vi "Upgrade to Secure Server VISA Socket.vi"(7 "immutable TLS Configuration":refnum<k36>, 8 "error in (no error)":errorcluster, 9 "timeout (5000ms)":i32=5000, 11 "VISA TCP Socket in":refnum<class "VISA TCP.lvclass">) -> (0 "error out":errorcluster, 2 "client certificate chain":cluster{"certificate":u8[]}[](array[cluster]), 3 "Secure Server VISA Socket out":refnum<class "VISA TCP.lvclass">)   [LabVIEW 2020, in "Secure Sockets Addon.lvlib"]
doc: "Upgrades a Server VISA TCP Socket to use TLS."
uses:
  Secure Sockets Addon.lvlib
  <vilib>/MediaMongrels Ltd/WebSockets/Sockets/VISA TCP Socket/VISA TCP.lvclass
  <vilib>/MediaMongrels Ltd/WebSockets/Sockets/VISA TCP Socket/VISA TCP.lvclass/VISA TCP.ctl
  <vilib>/MediaMongrels Ltd/WebSockets/Sockets/VISA TCP Socket/Read TCP Refnum.vi
  <vilib>/MediaMongrels Ltd/WebSockets/Sockets/VISA TCP Socket/Write TCP Refnum.vi
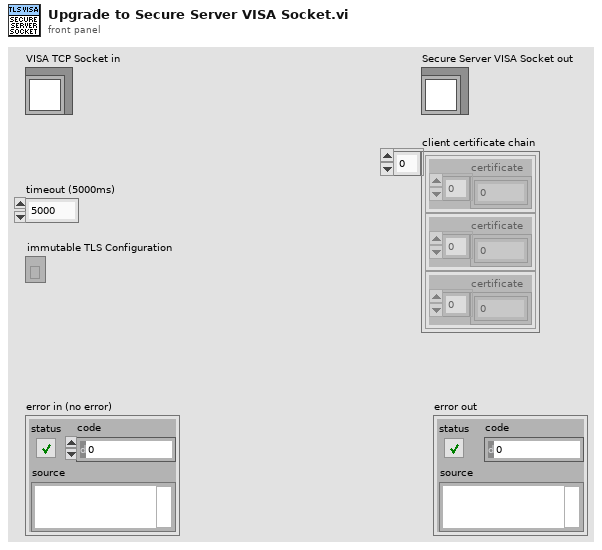
[diagram p1: front panel]
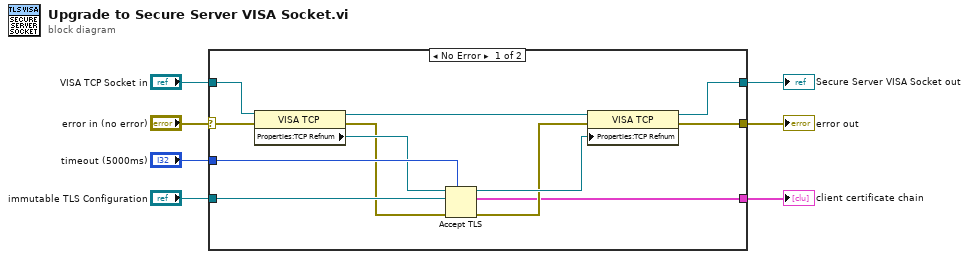
[diagram p0: block diagram]
diagram:
  n1 = case shown="No Error" "error in (no error)" {
    selector: "error in (no error)" -> [w12 w21]
    tunnel: "VISA TCP Socket in" -> [w19 w20]
    tunnel: "timeout (5000ms)" -> [w18 _]
    tunnel: [w14 w21] -> w5
    tunnel: [w13 w20] -> w4
    tunnel: "immutable TLS Configuration" -> [w10 _]
    tunnel: [w8 _] -> w1
    frame No Error {
      n2 = property class="VISA TCP"(reference=w19, error in=w12) -> (reference out=w16:refnum<class "VISA TCP.lvclass">, error out=w9:errorcluster, "Properties:TCP Refnum"=w11:refnum<k5>)
      n3 = Accept TLS(7:w18, 8:w9, 10:w10, 11:w11) -> (0:w15:errorcluster, 2:w8:cluster{"certificate":u8[]}[], 3:w17:refnum<k5>)
      n4 = property class="VISA TCP"(reference=w16, error in=w15, "Properties:TCP Refnum"=w17) -> (reference out=w13:refnum<class "VISA TCP.lvclass">, error out=w14:errorcluster)
    }
    frame Error {
    }
  }
  "error out" <- w5
  "Secure Server VISA Socket out" <- w4
  "client certificate chain" <- w1
